vi "Mars3D calibration check.vi"(4 "Numeric 3":i32, 5 "Right Eye in":T1, 6 "Numeric 2":i32, 7 "Numeric 6":i32, 8 "Left Eye in":T1, 9 "Numeric":i32, 10 "Numeric 4":i32, 11 "Numeric 5":i32) -> (0 "no calibration":bool, 2 "Left Eye out":T1, 3 "Right Eye out":T1)   [LabVIEW 2016]
panel:
  in  "Left Eye":T1 {"y" format="%.2f"; "z" format="%.2f"; "theta" format="%.2f"; "phi" format="%.2f"; "d" format="%.2f"}
  in  "Right Eye":T1 {"y" format="%.2f"; "z" format="%.2f"; "theta" format="%.2f"; "phi" format="%.2f"; "d" format="%.2f"}
  in  "OK Button":bool
  # "Calibration values missing. Please enter by hand"
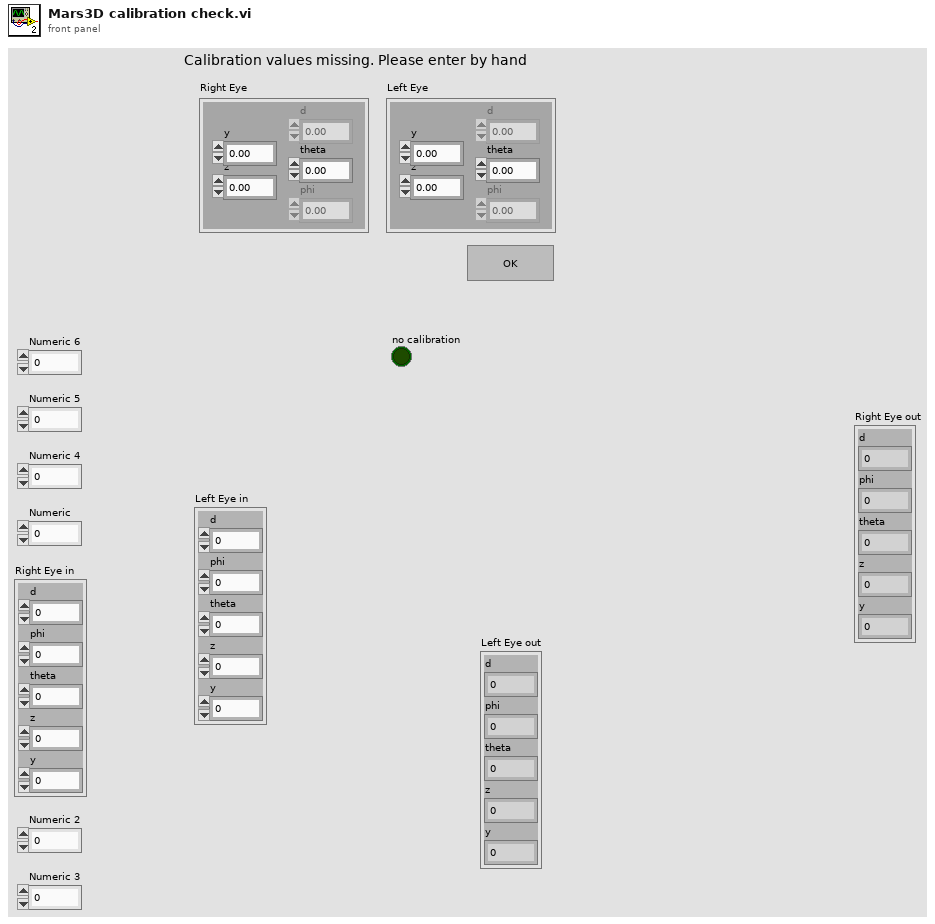
[diagram p1: front panel]
types:
  T1 = cluster{"d":dbl, "phi":dbl, "theta":dbl, "z":dbl, "y":dbl}
  T2 = enum32{"Invalid", "Standard", "Closed", "Hidden", "Minimized", "Maximized"}
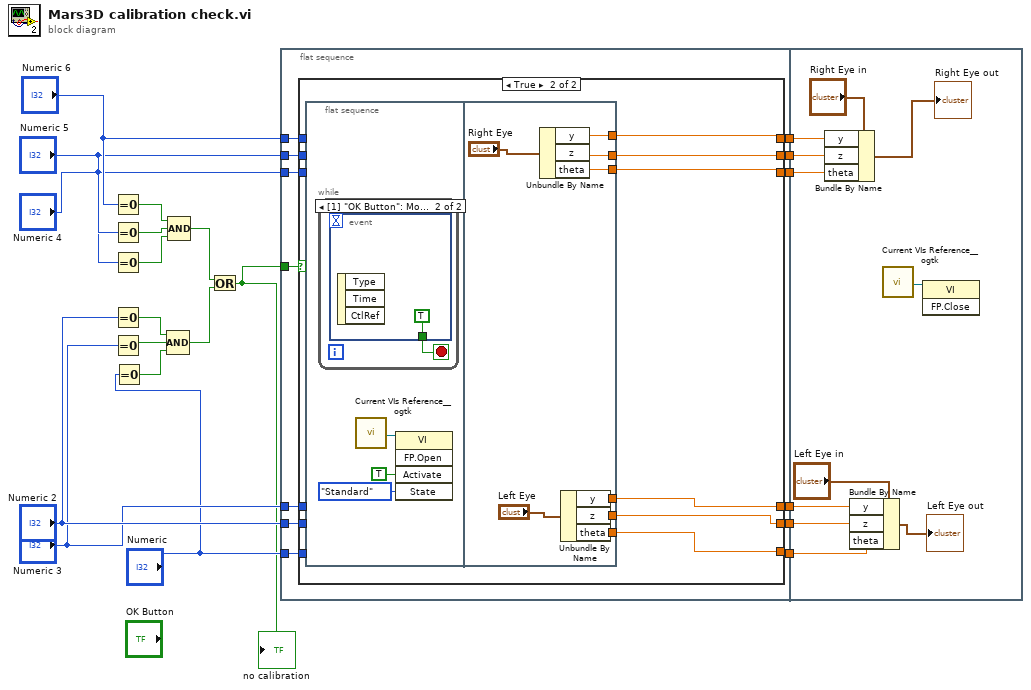
[diagram p0: block diagram]
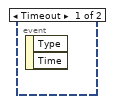
[diagram p3: hidden frame]
diagram:
  n1 = Equal To 0?(x="Numeric 6") -> (x = 0?=w15:bool)
  n2 = Equal To 0?(x="Numeric 5") -> (x = 0?=w14:bool)
  n3 = Equal To 0?(x="Numeric 4") -> (x = 0?=w13:bool)
  n4 = Equal To 0?(x="Numeric 2") -> (x = 0?=w12:bool)
  n5 = Equal To 0?(x="Numeric 3") -> (x = 0?=w11:bool)
  n6 = Equal To 0?(x="Numeric") -> (x = 0?=w10:bool)
  n7 = Compound Arithmetic op=AND(w12, w11, w10) -> (w8:bool)
  n8 = Compound Arithmetic op=AND(w15, w14, w13) -> (w9:bool)
  n9 = Or(x=w9, y=w8) -> (x .or. y?=w1:bool)
  "no calibration" <- w1
  n10 = flat-sequence {
    tunnel: "Numeric" -> [w22]
    tunnel: "Numeric 3" -> [w24]
    tunnel: "Numeric 2" -> [w23]
    tunnel: "Numeric 4" -> [w25]
    tunnel: "Numeric 5" -> [w26]
    tunnel: "Numeric 6" -> [w27]
    tunnel: [w33] -> w7
    tunnel: [w32] -> w6
    tunnel: [w31] -> w5
    tunnel: [w29] -> w4
    tunnel: [w30] -> w3
    tunnel: [w28] -> w2
    tunnel: w1 -> [w34]
    tunnel: w7 -> [w66]
    tunnel: w6 -> [w65]
    tunnel: w5 -> [w64]
    tunnel: w4 -> [w63]
    tunnel: w3 -> [w62]
    tunnel: w2 -> [w61]
    frame #0 {
      n11 = case shown="True" w34 {
        tunnel: [w40 w46] -> w33
        tunnel: [w39 w45] -> w32
        tunnel: [w38 w44] -> w31
        tunnel: [w37 w43] -> w30
        tunnel: [w36 w42] -> w29
        tunnel: [w35 w41] -> w28
        tunnel: w27 -> [w40 _]
        tunnel: w26 -> [w39 _]
        tunnel: w25 -> [w38 _]
        tunnel: w24 -> [w37 _]
        tunnel: w23 -> [w36 _]
        tunnel: w22 -> [w35 _]
        frame False {
        }
        frame True {
          n12 = flat-sequence {
            tunnel: [w57] -> w46
            tunnel: [w56] -> w45
            tunnel: [w55] -> w44
            tunnel: [w54] -> w43
            tunnel: [w53] -> w42
            tunnel: [w52] -> w41
            frame #0 {
              n13 = while {
                stop <- w50 stop-if-true
                n14 = event shown="[1] \"OK Button\": Mouse Up" {
                  selector: _ -> [_ _]
                  dyn-events: _ -> [_ _]
                  timeout: _ -> [_ _]
                  tunnel: [_ TRUE] -> w50
                  event Timeout {
                    n15 = event-data() -> ()  [unwired: 1 in, 2 out]
                  }
                  event "OK Button": Mouse Up {
                    n16 = event-data() -> ()  [unwired: 1 in, 3 out]
                  }
                }
              }
              n17 = call <userlib>:"Current VIs Reference__ogtk.vi"() -> ("Current VI's reference"=w47:refnum<vi>)  [unwired: 5 in]
              n18 = invoke class="VI" method="FP.Open"(reference=w47, "Activate"=TRUE ("Activate?"), "State"=T2."Standard") -> ()  [unwired: 2 in, 5 out]
            }
            frame #1 {
              n19 = Unbundle By Name("Right Eye") -> ("y"=w57:dbl, "z"=w56:dbl, "theta"=w55:dbl)
              n20 = Unbundle By Name("Left Eye") -> ("y"=w54:dbl, "z"=w53:dbl, "theta"=w52:dbl)
            }
          }
        }
      }
    }
    frame #1 {
      n21 = Bundle By Name(cluster="Right Eye in", "y"=w66, "z"=w65, "theta"=w64) -> (→"Right Eye out":T1)
      n22 = Bundle By Name(cluster="Left Eye in", "y"=w62, "z"=w63, "theta"=w61) -> (→"Left Eye out":T1)
      n23 = call <userlib>:"Current VIs Reference__ogtk.vi"() -> ("Current VI's reference"=w60:refnum<vi>)  [unwired: 5 in]
      n24 = invoke class="VI" method="FP.Close"(reference=w60) -> ()  [unwired: 2 in, 3 out]
    }
  }
